vi "Load and Build.vi"(0 "Project Path":path, 1 "Data String (\"\")":string, 5 "Report Folder":path, 7 "Build Config Override":path, 9 "Project Build Class Name (Empty = \"Project Builder\")":string, 11 "error in (no error)":errorcluster) -> (4 "Project Builder out":refnum<class "Project Builder.lvclass">, 10 "Success?":bool, 15 "error out":errorcluster)   [LabVIEW 2019, in "ProjectBuilder.lvlib"]
doc: "Load and populate a 'Project Builder'-class and call the Build Project.vi method on the loaded class."
uses:
  ProjectBuilder.lvlib
  PPL/HDH.ClassLoader.lvlibp
  Class/Project Builder/Project Builder.lvclass
  <vilib>/ErrorRing/Error Ring.xnode
  <vilib>/Utility/error.llb/Error Cluster From Error Code.vi
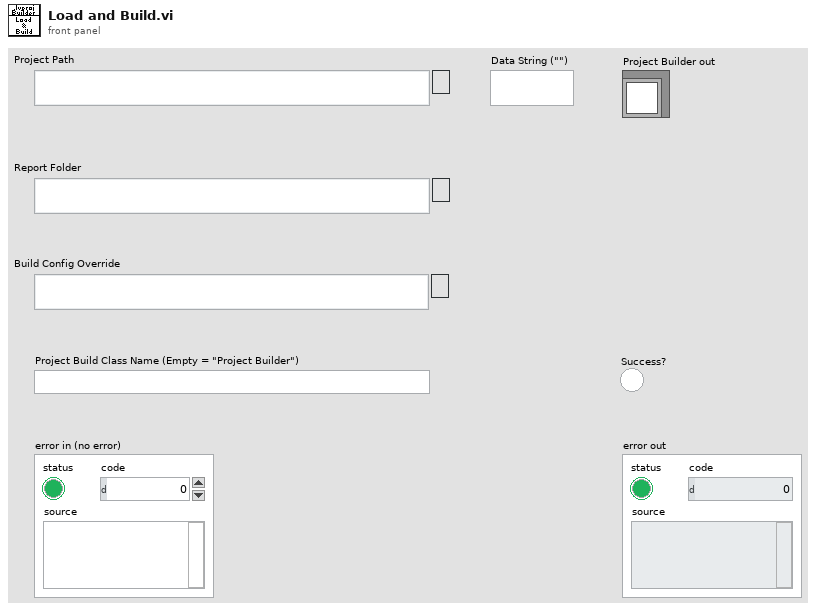
[diagram p1: front panel]
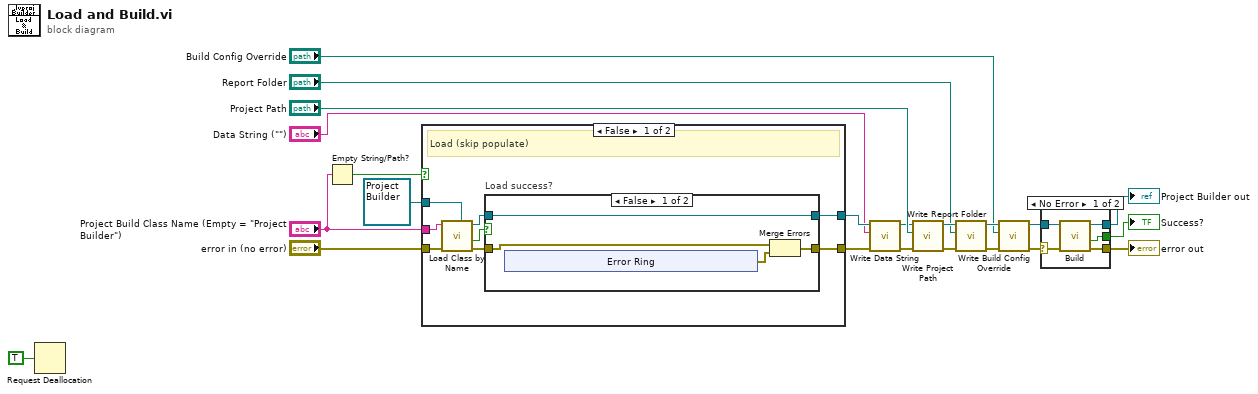
[diagram p0: block diagram]
diagram:
  n1 = Request Deallocation(TRUE ("flag")) -> ()
  n2 = Empty String/Path?(string/path="Project Build Class Name (Empty = \"Project Builder\")") -> (empty?=w22:bool)
  n3 = case shown="False" w22 {
    tunnel: "Project Build Class Name (Empty = \"Project Builder\")" -> [w30 _]
    tunnel: "error in (no error)" -> [w29 w41]
    tunnel: refnum<class "Project Builder.lvclass"> refnum ("ProjectBuilder.lvlib:Project Builder.lvclass") -> [w28 w42]
    tunnel: [w26 w42] -> w3
    tunnel: [w24 w41] -> w15
    frame False {
      # "Load (skip populate)"
      n4 = call "Load Class by Name.vi"("Class Type"=w28, "error in (no error)"=w29, "Base Class Name"=w30) -> ("error out"=w25:errorcluster, "Load and Type Success?"=w23:bool, "Loaded Class"=w27:refnum<class "Project Builder.lvclass">)  [unwired: 5 in, 1 out]
      n5 = case "Load success?" shown="False" w23 {
        tunnel: w27 -> [w34 w40]
        tunnel: [w34 w40] -> w26
        tunnel: w25 -> [w32 w39]
        tunnel: [w31 w39] -> w24
        frame False {
          n6 = xnode "Error Ring"() -> ("error out"=w33:errorcluster)
          n7 = Merge Errors(w32, w33) -> (w31:errorcluster)
        }
        frame True {
        }
      }
    }
    frame True {
      # "Use parent (don't populate)"
    }
  }
  n8 = call "Write Data String.vi"("error in (no error)"=w15, "Data"="Data String (\"\")", "Project Builder in"=w3) -> ("error out"=w4:errorcluster, "Project Builder out"=w2:refnum<class "Project Builder.lvclass">)  [unwired: 7 in]
  n9 = call "Write Project Path.vi"("error in (no error)"=w4, "Project Path"="Project Path", "Project Builder in"=w2) -> ("error out"=w14:errorcluster, "Project Builder out"=w18:refnum<class "Project Builder.lvclass">)  [unwired: 7 in]
  n10 = call "Write Report Folder.vi"("error in (no error)"=w14, "Report Folder"="Report Folder", "Project Builder in"=w18) -> ("error out"=w13:errorcluster, "Project Builder out"=w7:refnum<class "Project Builder.lvclass">)  [unwired: 7 in]
  n11 = call "Write Build Config Override.vi"("error in (no error)"=w13, "Build Config Override"="Build Config Override", "Project Builder in"=w7) -> ("error out"=w8:errorcluster, "Project Builder out"=w6:refnum<class "Project Builder.lvclass">)  [unwired: 7 in]
  n12 = case shown="No Error" w8 {
    selector: w8 -> [w46 w49]
    tunnel: w6 -> [w47 w48]
    tunnel: [w45 w49] -> w12
    tunnel: [w44 _] -> w11
    tunnel: [w43 w48] -> w10
    frame No Error {
      n13 = call "Build.vi"("error in (no error)"=w46, "Project Builder in"=w47) -> ("error out"=w45:errorcluster, "Success?"=w44:bool, "Project Builder out"=w43:refnum<class "Project Builder.lvclass">)  [unwired: 7 in]
    }
    frame Error {
    }
  }
  "error out" <- w12
  "Success?" <- w11
  "Project Builder out" <- w10
